vi "AddTwoNumbers.vi"(9 "Numeric 2":dbl, 11 "Numeric":dbl) -> (3 "Sum":dbl)   [LabVIEW 2013, in "CustomProjectLibrary.lvlib"]
uses:
  CustomProjectLibrary.lvlib
  <vilib>/express/express arith-compare/Formula/XNode/ExpressFormulaBlockNode.xnode
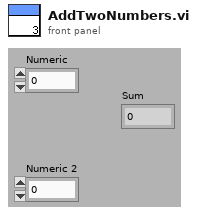
[diagram p1: front panel]
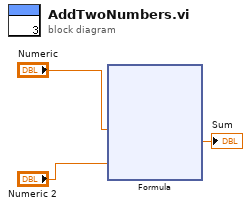
[diagram p0: block diagram]
diagram:
  n1 = xnode "Formula"("X1"="Numeric", "X2"="Numeric 2") -> ("Result"=→"Sum":dbl)  [unwired: 1 in, 1 out]
